vi "Shooter Gathering Velocity.vi"() -> ()   [LabVIEW 2011]
panel:
  in  "Shooter Gathering Velocity":dbl=-6000.0
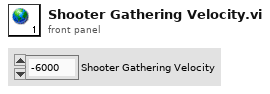
[diagram p1: front panel]
diagram:
